vi "Move Job Files to Workspace.vi"(8 "error in (no error)":errorcluster, 10 "Generated Files":path[](array[path]), 11 "Workspace Path":string) -> (0 "error out":errorcluster)   [LabVIEW 2014, in "lv-cli-steps.lvlib"]
uses:
  lv-cli-steps.lvlib
panel:
  # "Input"
  # "Output"
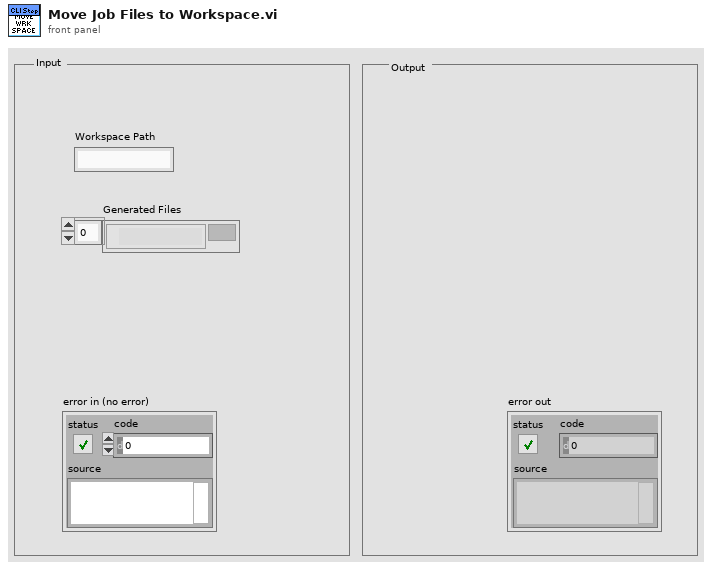
[diagram p1: front panel]
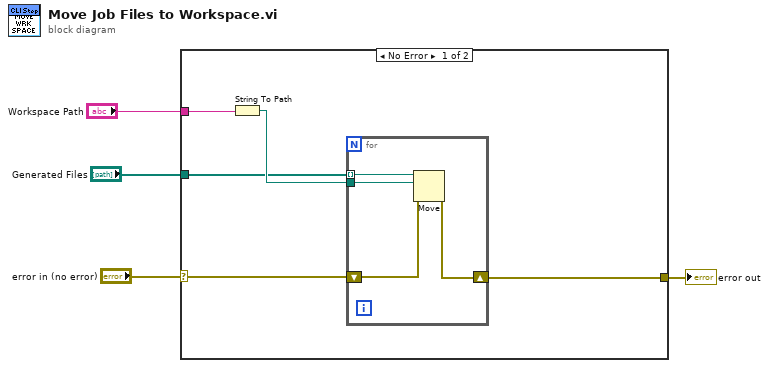
[diagram p0: block diagram]
diagram:
  n1 = case shown="No Error" "error in (no error)" {
    selector: "error in (no error)" -> [w6 w14]
    tunnel: "Workspace Path" -> [w9 _]
    tunnel: "Generated Files" -> [w7 _]
    tunnel: [w5 w14] -> w1
    frame No Error {
      n2 = String To Path(string=w9) -> (path=w8:path)
      n3 = for {
        tunnel: w8 -> [w13]
        tunnel: w7 -> [w12] mode=indexing
        shift-right: [w10] -> w5
        shift-left: w6 -> [w11]
        n4 = Move(source path=w12, error in=w11, 10:w13) -> (error out=w10:errorcluster)  [unwired: 2 in, 2 out]
      }
    }
    frame Error {
    }
  }
  "error out" <- w1
